vi "TUNA at the waypoint.vi"(1 "Y location":dbl, 2 "X location":dbl, 3 "Yof waypoint":dbl, 4 "X of waypoint":dbl) -> (0 "At Waypoint?":bool)   [LabVIEW 2014]
doc: "This VI calculates the distance between the boat and a waypoint. If they are within 60 pixels the boat is at the waypoint. The output is Yes or No."
panel:
  in  "Radius":dbl=10.0 format="%#_13g"
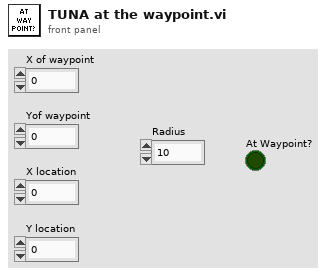
[diagram p1: front panel]
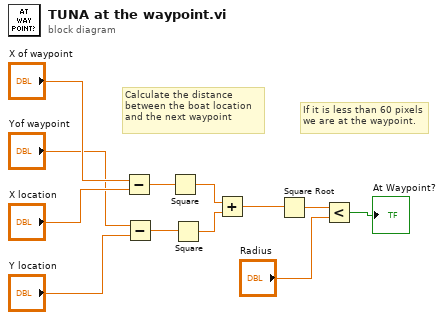
[diagram p0: block diagram]
diagram:
  # "If it is less than 60 pixels\nwe are at the waypoint."
  # "Calculate the distance\nbetween the boat location\nand the next waypoint"
  n1 = Subtract(x="X of waypoint", y="X location") -> (x-y=w12:dbl)
  n2 = Subtract(x="Yof waypoint", y="Y location") -> (x-y=w11:dbl)
  n3 = Square(x=w12) -> (x^2=w10:dbl)
  n4 = Square(x=w11) -> (x^2=w9:dbl)
  n5 = Add(x=w10, y=w9) -> (x+y=w1:dbl)
  n6 = Square Root(x=w1) -> (sqrt(x)=w8:dbl)
  n7 = Less?(x=w8, y="Radius") -> (x < y?=→"At Waypoint?":bool)
